vi "Main_Log_Queue.vi"(0 "Generated_Data_In":T1, 11 "Error_In":errorcluster, 13 "Operation":T2=enum."Enqueue") -> (4 "Generated_Data_Out":T1, 6 "Generated_Data_Preview":T1[](array[typedef]), 8 "Overflow":bool, 10 "Underflow":bool, 15 "Error_Out":errorcluster)   [LabVIEW 2023]
doc: "It is a queue used to send data to other VIs or loops."
uses:
  Controls/Operation_Select_Queue.ctl
  Controls/Data.ctl
  Controls/Queue_and_Parameter.ctl
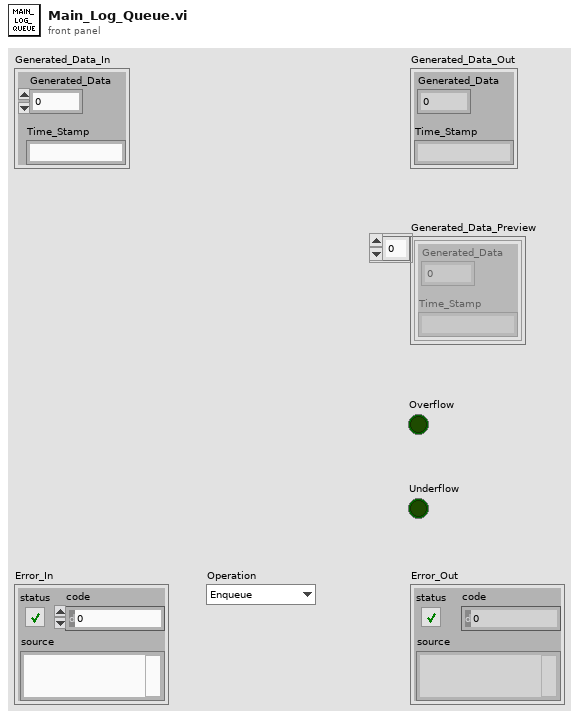
[diagram p1: front panel]
types:
  T1 = typedef "Data.ctl" = cluster{"Generated_Data":dbl, "Time_Stamp":string}
  T2 = typedef "Operation_Select_Queue.ctl" = enum16{"Initialize", "Enqueue", "Dequeue", "Preview"}
  T3 = typedef "Queue_and_Parameter.ctl" = cluster{"Head_Pointer":i32, "Dimention_Size":i32, "Data":T1[]}
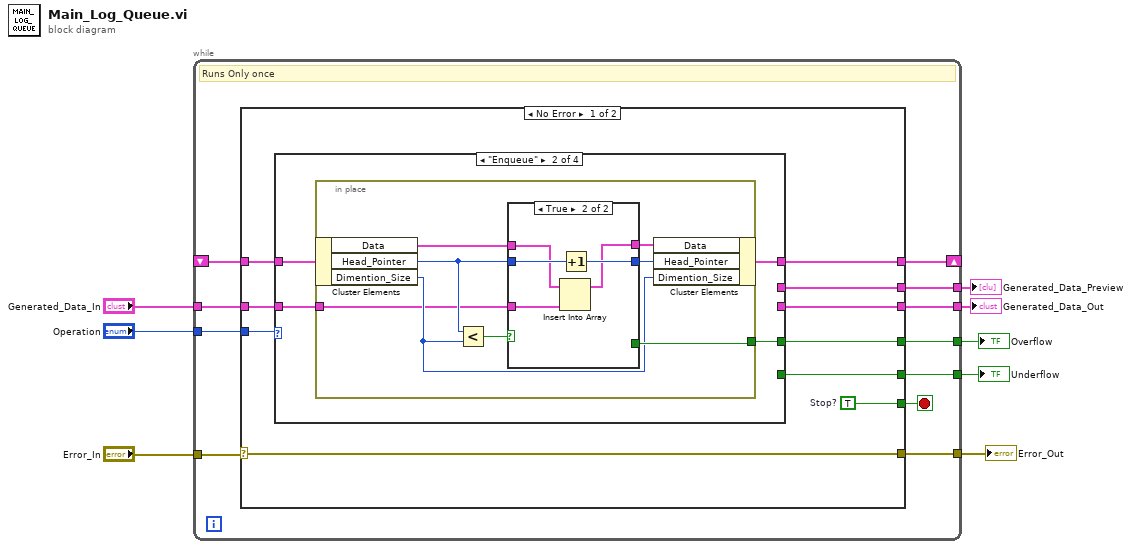
[diagram p0: block diagram]
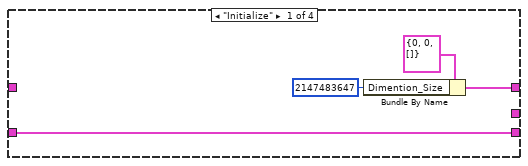
[diagram p2: hidden frame]
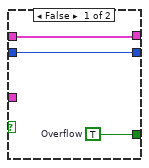
[diagram p3: hidden frame]
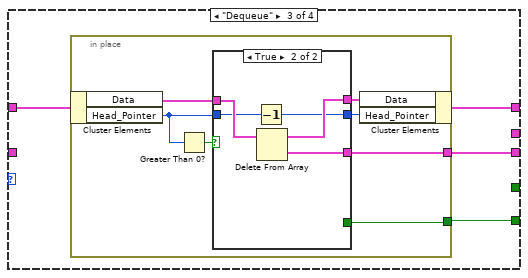
[diagram p4: hidden frame]
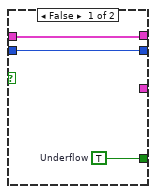
[diagram p5: hidden frame]
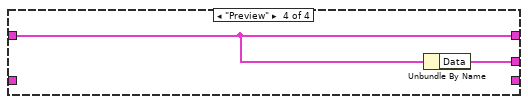
[diagram p6: hidden frame]
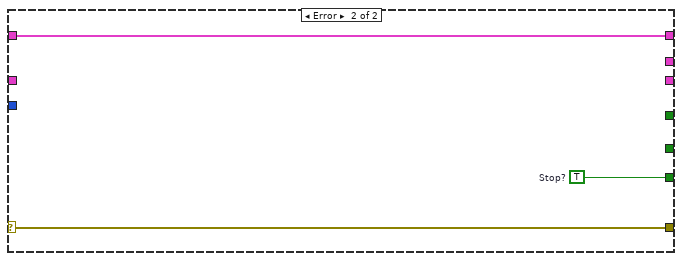
[diagram p7: hidden frame]
diagram:
  n1 = while {
    tunnel: [w19] -> w2
    tunnel: "Operation" -> [w18]
    tunnel: [w16] -> w7
    tunnel: [w15] -> w6
    shift-right: [w14] -> _
    shift-left: _ -> [w13]
    tunnel: "Error_In" -> [w12]
    tunnel: [w11] -> w4
    tunnel: [w10] -> w1
    tunnel: "Generated_Data_In" -> [w9]
    stop <- w17 stop-if-true
    # "Runs Only once"
    n2 = case shown="No Error" w12 {
      selector: w12 -> [w22 w75]
      tunnel: [w29 _] -> w19
      tunnel: w18 -> [w28 _]
      tunnel: [w27 w76] -> w17
      tunnel: [w26 _] -> w16
      tunnel: [w25 _] -> w15
      tunnel: [w24 w77] -> w14
      tunnel: w13 -> [w23 w77]
      tunnel: [w22 w75] -> w11
      tunnel: [w21 _] -> w10
      tunnel: w9 -> [w20 _]
      frame No Error {
        w27 = TRUE  # Stop?
        n3 = case shown="\"Enqueue\"" w28 {
          tunnel: w23 -> [_ w36 w54 w74]
          tunnel: [w30 _ w57 _] -> w29
          tunnel: [_ w37 _ _] -> w26
          tunnel: [_ _ w56 _] -> w25
          tunnel: [w33 w35 w55 w74] -> w24
          tunnel: [_ _ _ w73] -> w21
          tunnel: w20 -> [w30 w34 _ _]
          frame "Initialize" {
            n4 = Bundle By Name(cluster=T3 {"Head_Pointer"=0, "Dimention_Size"=0, "Data"=[]}, "Dimention_Size"=2147483647) -> (w33:T3)
          }
          frame "Enqueue" {
            n5 = in-place "In Place Element Structure" {
              in-place-border: [w44] -> w37
              in-place-border: w34 -> [w38]
              n6 = in-place-cluster #1(w36) -> ("Data"=w43:T1[], "Head_Pointer"=w40:i32, "Dimention_Size"=w39:i32)
              n7 = Less?(x=w40, y=w39) -> (x < y?=w45:bool)
              n8 = case shown="True" w45 {
                tunnel: w43 -> [w47 w50]
                tunnel: [w47 w51] -> w41
                tunnel: w40 -> [w48 w53]
                tunnel: [w48 w52] -> w42
                tunnel: [w46 _] -> w44
                tunnel: w38 -> [_ w49]
                frame False {
                  w46 = TRUE  # Overflow
                }
                frame True {
                  n9 = Insert Into Array(array=w50, new element=w49) -> (w51:T1[])  [unwired: 1 in]
                  n10 = Increment(x=w53) -> (x+1=w52:i32)
                }
              }
              n11 = in-place-cluster #1("Data"=w41, "Head_Pointer"=w42, "Dimention_Size"=w39) -> (w35:T3)
            }
          }
          frame "Dequeue" {
            n12 = in-place "In Place Element Structure" {
              in-place-border: [w64] -> w57
              in-place-border: [w62] -> w56
              n13 = in-place-cluster #2(w54) -> ("Data"=w59:T1[], "Head_Pointer"=w60:i32)
              n14 = Greater Than 0?(x=w60) -> (x > 0?=w61:bool)
              n15 = case shown="True" w61 {
                tunnel: [w67 w71] -> w58
                tunnel: w59 -> [w67 w72]
                tunnel: [_ w70] -> w64
                tunnel: w60 -> [w66 w69]
                tunnel: [w66 w68] -> w63
                tunnel: [w65 _] -> w62
                frame False {
                  w65 = TRUE  # Underflow
                }
                frame True {
                  n16 = Decrement(x=w69) -> (x-1=w68:i32)
                  n17 = Delete From Array(array=w72) -> (deleted portion=w70:T1, array with subset deleted=w71:T1[])  [unwired: 2 in]
                }
              }
              n18 = in-place-cluster #2("Data"=w58, "Head_Pointer"=w63) -> (w55:T3)
            }
          }
          frame "Preview" {
            n19 = Unbundle By Name(w74) -> ("Data"=w73:T1[])
          }
        }
      }
      frame Error {
        w76 = TRUE  # Stop?
      }
    }
  }
  "Error_Out" <- w4
  "Overflow" <- w7
  "Underflow" <- w6
  "Generated_Data_Out" <- w2
  "Generated_Data_Preview" <- w1
